vi "actuate_voltageStepExp_v0.05.vi"(0 "Phase Cluster":T4, 1 "valve Time Cluster":T3, 2 "Didn't Lift?":bool, 3 "data in":T5={"daq_ao 1"="Dev1/ao0", "daq_ai 1"="Dev1/ai0", "experiment day folder"=path "D:/DATA/8-27-15 save func testing/test.lvm", "Multiclamp init error"=0, "Multiclamp Handle Out"=0, "sampling rate (Hz)"=10000, "trial name"=""}, 5 "PhaseLetter":string, 7 "controls array in":refnum<vi>[](array[refnum]), 9 "time to wait for solution change (min)":dbl=2.5 min=0.0 step=0.01, 11 "error in":errorcluster, 12 "common cluster":T7, 13 "individual controls in":T6) -> (4 "output cluster":T1, 6 "protocol waveform":waveform(dbl)[](graph), 8 "jumptestMonitor":waveform(dbl)[](graph) caption="protocol response", 10 "control array out":refnum<vi>[](array[refnum]), 14 "experiment VI ref":refnum<vi>, 15 "error out":errorcluster)   [LabVIEW 2019]
uses:
  pipette cleaning/pressure box/cleaning_soft/controls/actuator_type.ctl
  pipette cleaning/pressure box/cleaning_soft/controls/actuator_cluster.ctl
  machine_vision/coordinate model vis/transform_properties_actuators.ctl
  machine_vision/controls/transform_cluster_actuator.ctl
  controls/NH_method.ctl
  pipette cleaning/pressure box/cleaning_soft/controls/pressure_box_type.ctl
  pipette cleaning/pressure box/cleaning_soft/controls/pressure_box_control.ctl
  multipatch/controls/multipatch_common_controls_v4.ctl
  controls/memtest_def.ctl
  multipatch/controls/multipatch_individual_controls_v5.ctl
  Controls/Data.ctl
panel:
  in  "VoltageStepValuesCluster":T2
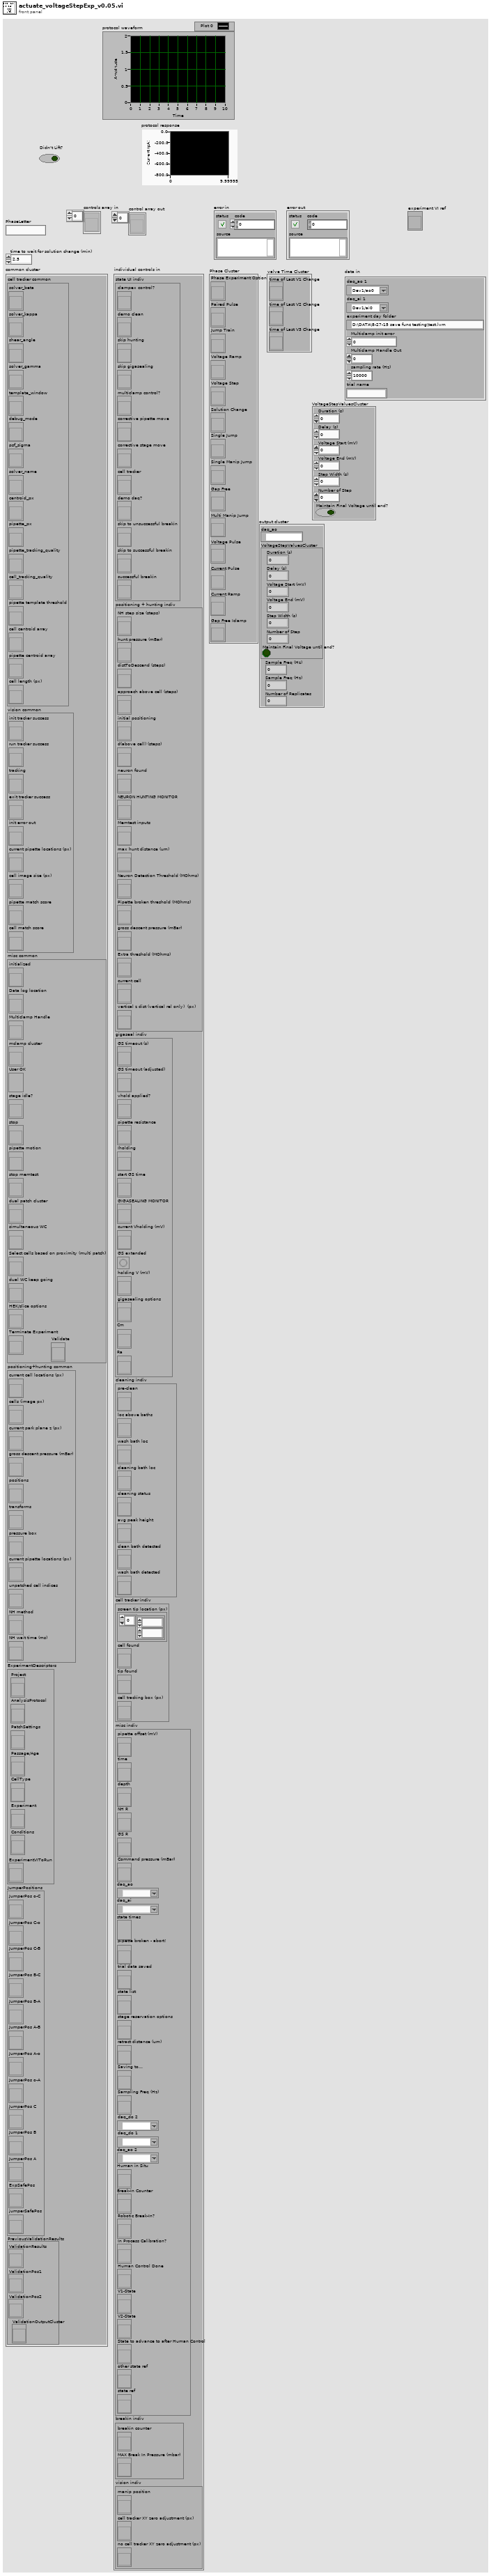
[diagram p1: front panel]
types:
  T1 = cluster{"daq_ao":tag, "VoltageStepValuesCluster":cluster{"Duration (s)":dbl, "Delay (s)":dbl, "Voltage Start (mV)":dbl, "Voltage End (mV)":dbl, "Step Width (s)":dbl, "Number of Step":dbl, "Maintain Final Voltage until end?":bool}, "Sample Freq (Hz)":dbl, "Sample Freq (Hz)":dbl, "Number of Replicates":i16}
  T2 = cluster{"Duration (s)":dbl, "Delay (s)":dbl, "Voltage Start (mV)":dbl, "Voltage End (mV)":dbl, "Step Width (s)":dbl, "Number of Step":dbl, "Maintain Final Voltage until end?":bool}
  T3 = cluster{"time of Last V1 Change":refnum<vi>, "time of Last V2 Change":refnum<vi>, "time of Last V3 Change":refnum<vi>}
  T4 = cluster{"Phase Experiment Option":refnum<vi>, "Paired Pulse":refnum<vi>, "Jump Train":refnum<vi>, "Voltage Ramp":refnum<vi>, "Voltage Step":refnum<vi>, "Solution Change":refnum<vi>, "Single Jump":refnum<vi>, "Single Manip Jump":refnum<vi>, "Gap Free":refnum<vi>, "Multi Manip Jump":refnum<vi>, "Voltage Pulse":refnum<vi>, "Current Pulse":refnum<vi>, "Current Ramp":refnum<vi>, "Gap Free Iclamp":refnum<vi>}
  T5 = typedef "Data.ctl" = cluster{"daq_ao 1":tag, "daq_ai 1":tag, "experiment day folder":path, "Multiclamp init error":i32, "Multiclamp Handle Out":u32, "sampling rate (Hz)":i32, "trial name":string}
  T6 = typedef "multipatch_individual_controls_v5.ctl" = cluster{"state UI indiv":cluster{"clampex control?":refnum<vi>, "demo clean":refnum<vi>, "skip hunting":refnum<vi>, "skip gigasealing":refnum<vi>, "multiclamp control?":refnum<vi>, "corrective pipette move":refnum<vi>, "corrective stage move":refnum<vi>, "cell tracker":refnum<vi>, "demo daq?":refnum<vi>, "skip to unsuccessful breakin":refnum<vi>, "skip to successful breakin":refnum<vi>, "successful breakin":refnum<vi>}, "positioning + hunting indiv":cluster{"NH step size (steps)":refnum<vi>, "hunt pressure (mBar)":refnum<vi>, "distToDescend (steps)":refnum<vi>, "approach above cell (steps)":refnum<vi>, "initial positioning":refnum<vi>, "d(above cell) (steps)":refnum<vi>, "neuron found":refnum<vi>, "NEURON HUNTING MONITOR":refnum<vi>, "Memtest inputs":refnum<vi>, "max hunt distance (um)":refnum<vi>, "Neuron Detection Threshold (MOhms)":refnum<vi>, "Pipette broken threshold (MOhms)":refnum<vi>, "gross descent pressure (mBar)":refnum<vi>, "Extra threshold (MOhms)":refnum<vi>, "current cell":refnum<vi>, "vertical z dist (vertical rel only)  (px)":refnum<vi>}, "gigaseal indiv":cluster{"GS timeout (s)":refnum<vi>, "GS timeout (adjusted)":refnum<vi>, "vhold applied?":refnum<vi>, "pipette resistance":refnum<vi>, "Iholding":refnum<vi>, "start GS time":refnum<vi>, "GIGASEALING MONITOR":refnum<vi>, "current Vholding (mV)":refnum<vi>, "GS extended":refnum<vi>, "holding V (mV)":refnum<vi>, "gigasealing options":refnum<vi>, "Cm":refnum<vi>, "Ra ":refnum<vi>}, "cleaning indiv":cluster{"pre-clean":refnum<vi>, "loc above baths":refnum<vi>, "wash bath loc":refnum<vi>, "cleaning bath loc":refnum<vi>, "cleaning status":refnum<vi>, "avg peak height":refnum<vi>, "clean bath detected":refnum<vi>, "wash bath detected":refnum<vi>}, "cell tracker indiv":cluster{"screen tip location (px)":refnum<vi>, "cell found":refnum<vi>, "tip found":refnum<vi>, "cell tracking box (px)":refnum<vi>}, "misc indiv":cluster{"pipette offset (mV)":refnum<vi>, "time":refnum<vi>, "depth":refnum<vi>, "NH R":refnum<vi>, "GS R":refnum<vi>, "Command pressure (mBar)":refnum<vi>, "daq_ao":tag, "daq_ai":tag, "state times":refnum<vi>, "pipette broken - abort!":refnum<vi>, "trial data saved":refnum<vi>, "state list":refnum<vi>, "stage reservation options":refnum<vi>, "retract distance (um)":refnum<vi>, "Saving to...":refnum<vi>, "Sampling Freq (Hz)":refnum<vi>, "daq_do 2":tag, "daq_do 1":tag, "daq_ao 2":tag, "Human in Situ":refnum<vi>, "Break-In Counter":refnum<vi>, "Robotic Break-In?":refnum<vi>, "In Process Calibration?":refnum<vi>, "Human Control Done":refnum<vi>, "V1-State":refnum<vi>, "V2-State":refnum<vi>, "State to advance to after Human Control":refnum<vi>, "other state ref":refnum<vi>, "state ref":refnum<vi>}, "breakin indiv":cluster{"breakin counter":refnum<vi>, "MAX Break In Pressure (mbar)":refnum<vi>}, "vision indiv":cluster{"manip position":refnum<vi>, "cell tracker XY zero adjustment (px)":refnum<vi>, "no cell tracker XY zero adjustment (px)":refnum<vi>}}
  T7 = typedef "multipatch_common_controls_v4.ctl" = cluster{"cell tracker common":cluster{"solver_beta":refnum<vi>, "solver_kappa":refnum<vi>, "shear_angle":refnum<vi>, "solver_gamma":refnum<vi>, "template_window":refnum<vi>, "debug_mode":refnum<vi>, "psf_sigma":refnum<vi>, "solver_name":refnum<vi>, "centroid_px":refnum<vi>, "pipette_px":refnum<vi>, "pipette_tracking_quality":refnum<vi>, "cell_tracking_quality":refnum<vi>, "pipette template threshold":refnum<vi>, "cell centroid array":refnum<vi>, "pipette centroid array":refnum<vi>, "cell length (px)":refnum<vi>}, "vision common":cluster{"init tracker success":refnum<vi>, "run tracker success":refnum<vi>, "tracking":refnum<vi>, "exit tracker success":refnum<vi>, "init error out":refnum<vi>, "current pipette locations (px)":refnum<vi>, "cell image size (px)":refnum<vi>, "pipette match score":refnum<vi>, "cell match score":refnum<vi>}, "misc common":cluster{"initialized":refnum<vi>, "Data log location":refnum<vi>, "Multiclamp Handle":refnum<vi>, "mclamp cluster":refnum<vi>, "User OK":refnum<vi>, "stage idle?":refnum<vi>, "stop":refnum<vi>, "pipette motion":refnum<vi>, "stop memtest":refnum<vi>, "dual patch cluster":refnum<vi>, "simultaneous WC":refnum<vi>, "Select cells based on proximity (multi patch)":refnum<vi>, "dual WC keep going":refnum<vi>, "HEK/slice options":refnum<vi>, "Terminate Experiment":refnum<vi>, "Validate":refnum<vi>}, "positioning+hunting common":cluster{"current cell locations (px)":refnum<vi>, "cells (image px)":refnum<vi>, "current park plane z (px)":refnum<vi>, "gross descent pressure (mBar)":refnum<vi>, "positions":refnum<vi>, "transforms":refnum<vi>, "pressure box":refnum<vi>, "current pipette locations (px)":refnum<vi>, "unpatched cell indices":refnum<vi>, "NH method":refnum<vi>, "NH wait time (ms)":refnum<vi>}, "ExperimentDescriptors":cluster{"Project":refnum<vi>, "AnalysisProtocol":refnum<vi>, "PatchSettings":refnum<vi>, "Passage/Age":refnum<vi>, "CellType":refnum<vi>, "Experiment":refnum<vi>, "Conditions":refnum<vi>, "ExperimentVIToRun":refnum<vi>}, "JumperPositions":cluster{"JumperPos o-C":refnum<vi>, "JumperPos C-o":refnum<vi>, "JumperPos C-B":refnum<vi>, "JumperPos B-C":refnum<vi>, "JumperPos B-A":refnum<vi>, "JumperPos A-B":refnum<vi>, "JumperPos A-o":refnum<vi>, "JumperPos o-A":refnum<vi>, "JumperPos C":refnum<vi>, "JumperPos B":refnum<vi>, "JumperPos A":refnum<vi>, "ExpSafePos":refnum<vi>, "jumperSafePos":refnum<vi>}, "PreviousValidationResults":cluster{"ValidationResults":refnum<vi>, "ValidationPos1":refnum<vi>, "ValidationPos2":refnum<vi>, "ValidationOutputCluster":refnum<vi>}}
  T8 = cluster{"Which Position to use for Experiment":enum16{"Jumper Safe Position", "Experiment Safe Position", "Jumper Position A", "Jumper Position B", "Jumper Position C", "Jumper Position o-A", "Jumper Position A-o", "Jumper Position A-B", "Jumper Position B-A", "Jumper Position B-C", "Jumper Position C-B", "Jumper Position C-o", "Jumper Position o-C", "Don't Move"}, "Duration (s)":dbl, "Delay (s)":dbl, "Step Width (s)":dbl, "Voltage Start (mV)":dbl, "Voltage Step (mV)":dbl, "Replicates":dbl, "Voltage End (mV)":dbl, "Number of Step":dbl, "Vholding (mV)":dbl, "Valve 1 Position":i16, "Valve 2 Position":i16, "Valve 3 Position":i16, "valve 1 used now?":bool, "valve 2 used now?":bool, "valve 3 used now? ":bool, "Total Step Time (s)":dbl, "Maintain Final Voltage until end?":bool, "protocol Preview":waveform(dbl)[]}
  T9 = enum16{"Jumper Safe Position", "Experiment Safe Position", "Jumper Position A", "Jumper Position B", "Jumper Position C", "Jumper Position o-A", "Jumper Position A-o", "Jumper Position A-B", "Jumper Position B-A", "Jumper Position B-C", "Jumper Position C-B", "Jumper Position C-o", "Jumper Position o-C", "Don't Move"}
  T10 = enum16{"manipulator 1", "manipulator 2", "manipulator 3", "manipulator 4"}
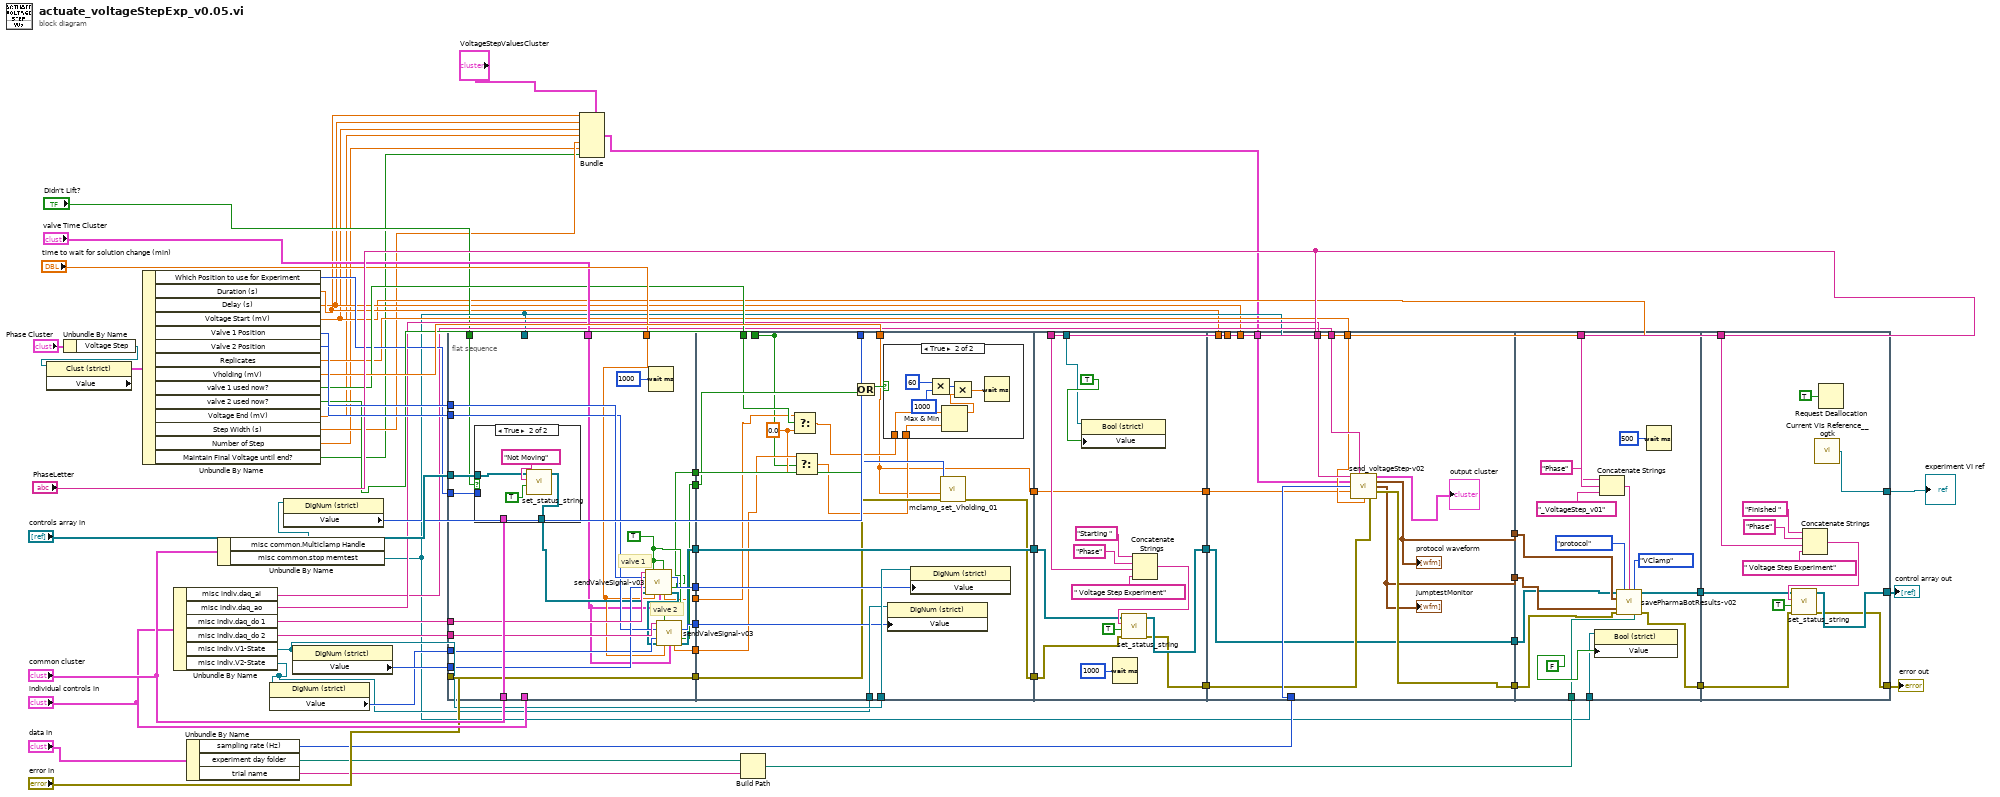
[diagram p0: block diagram]
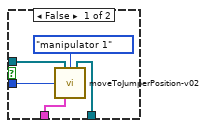
[diagram p2: hidden frame]
diagram:
  n1 = Unbundle By Name("Phase Cluster") -> ("Voltage Step"=w44:refnum<vi>)
  n2 = property class="Clust (strict)"(reference=w44) -> ("Value"=w43:T8)  [unwired: 1 in, 2 out]
  n3 = Unbundle By Name(w43) -> ("Which Position to use for Experiment"=w19:T9, "Duration (s)"=w12:dbl, "Delay (s)"=w11:dbl, "Voltage Start (mV)"=w10:dbl, "Valve 1 Position"=w42:i16, "Valve 2 Position"=w41:i16, "Replicates"=w18:dbl, "Vholding (mV)"=w28:dbl, "valve 1 used now?"=w21:bool, "valve 2 used now?"=w20:bool, "Voltage End (mV)"=w9:dbl, "Step Width (s)"=w8:dbl, "Number of Step"=w4:dbl, "Maintain Final Voltage until end?"=w3:bool)
  n4 = Unbundle By Name("individual controls in") -> ("misc indiv.daq_ai"=w15:tag, "misc indiv.daq_ao"=w16:tag, "misc indiv.daq_do 1"=w64:tag, "misc indiv.daq_do 2"=w63:tag, "misc indiv.V1-State"=w55:refnum<vi>, "misc indiv.V2-State"=w54:refnum<vi>)
  n5 = Unbundle By Name("data in") -> ("sampling rate (Hz)"=w17:i32, "experiment day folder"=w48:path, "trial name"=w47:string)
  n6 = Unbundle By Name("common cluster") -> ("misc common.Multiclamp Handle"=w27:refnum<vi>, "misc common.stop memtest"=w14:refnum<vi>)
  n7 = property class="DigNum (strict)"(reference=w54) -> ("Value"=w56:u16)  [unwired: 1 in, 2 out]
  n8 = property class="DigNum (strict)"(reference=w27) -> ("Value"=w26:u32)  [unwired: 1 in, 2 out]
  n9 = property class="DigNum (strict)"(reference=w55) -> ("Value"=w57:u16)  [unwired: 1 in, 2 out]
  n10 = flat-sequence {
    tunnel: "common cluster" -> [w89]
    tunnel: "individual controls in" -> [_]
    tunnel: [w86] -> w59
    tunnel: [w83] -> w53
    tunnel: [w82] -> w52
    tunnel: [w76] -> w35
    tunnel: [w74] -> w30
    tunnel: [w73] -> w29
    tunnel: "time to wait for solution change (min)" -> [w72]
    tunnel: "valve Time Cluster" -> [w71]
    tunnel: [w70] -> w23
    tunnel: [w69] -> w22
    tunnel: w14 -> [_]
    tunnel: "Didn't Lift?" -> [w67]
    tunnel: w19 -> [w90]
    tunnel: w64 -> [w88]
    tunnel: w63 -> [w87]
    tunnel: "error in" -> [w86]
    tunnel: w57 -> [w85]
    tunnel: w56 -> [w84]
    tunnel: w42 -> [w81]
    tunnel: w41 -> [w80]
    tunnel: "controls array in" -> [w79]
    tunnel: [w108] -> w60
    tunnel: w59 -> [w110]
    tunnel: w55 -> [w118]
    tunnel: w54 -> [w117]
    tunnel: w53 -> [w116]
    tunnel: w52 -> [w115]
    tunnel: [w114] -> w36
    tunnel: w35 -> [w114]
    tunnel: w30 -> [w112]
    tunnel: w29 -> [w111]
    tunnel: w28 -> [w100]
    tunnel: w26 -> [w109]
    tunnel: w23 -> [w105]
    tunnel: w22 -> [w104]
    tunnel: w21 -> [w106]
    tunnel: [w101] -> _
    tunnel: w20 -> [w101]
    tunnel: [w100] -> w5
    tunnel: w14 -> [w127]
    tunnel: [w129] -> w61
    tunnel: w60 -> [w130]
    tunnel: [w131] -> w37
    tunnel: w36 -> [w132]
    tunnel: "PhaseLetter" -> [w133]
    tunnel: [w126] -> w6
    tunnel: w5 -> [w126]
    tunnel: w15 -> [w151]
    tunnel: w16 -> [w150]
    tunnel: w61 -> [w145]
    tunnel: [w148] -> w51
    tunnel: [w142] -> w50
    tunnel: w18 -> [w146]
    tunnel: w12 -> [_]
    tunnel: w17 -> [w147]
    tunnel: w10 -> [_]
    tunnel: w11 -> [_]
    tunnel: [w144] -> w40
    tunnel: [w143] -> w38
    tunnel: w37 -> [w143]
    tunnel: w7 -> [w141]
    tunnel: w6 -> [w140]
    tunnel: w14 -> [w166]
    tunnel: w51 -> [w165]
    tunnel: w50 -> [w164]
    tunnel: w46 -> [w161]
    tunnel: "PhaseLetter" -> [w159]
    tunnel: w40 -> [w156]
    tunnel: w38 -> [w155]
    tunnel: [w153] -> w33
    tunnel: [w154] -> w32
    tunnel: [w173] -> w34
    tunnel: [w172] -> w58
    tunnel: w33 -> [w171]
    tunnel: w32 -> [w174]
    tunnel: "PhaseLetter" -> [w170]
    tunnel: [w169] -> w1
    frame #0 {
      w75 = TRUE ("Set Status")
      # "valve 2"
      # "valve 1"
      n11 = case shown="True" w67 {
        tunnel: w90 -> [w95 _]
        tunnel: w89 -> [w94 _]
        tunnel: w79 -> [w92 w96]
        tunnel: [w91 w97] -> w78
        frame False {
          n12 = call "moveToJumperPosition-v02.vi"("which manipulator"=T10."manipulator 1", "controls array in"=w92, "Which Jumper Position to move to?"=w95, "common cluster"=w94) -> ("control array out"=w91:refnum<vi>[])  [unwired: 10 in, 1 out]
        }
        frame True {
          n13 = call "set_status_string.vi"("new line?"=TRUE, "status string in"="Not Moving", "controls array"=w96) -> ("controls array out"=w97:refnum<vi>[])  [unwired: 7 in, 1 out]
        }
      }
      n14 = call "sendValveSignal-v03.vi"("daq_do"=w88, "Set Status"=w75, "Valve1?"=w75, "ChangeToValve"=w81, "CurrentValve"=w85, "controls array in"=w78, "time to wait for solution change (min)"=w72, "valve Time Cluster"=w71) -> ("ValveSetTo"=w82:u16, "valve changed?"=w74:bool, "additional time to wait (min)"=w70:dbl, "control array out"=w77:refnum<vi>[])  [unwired: 4 in]
      n15 = Wait (ms)(milliseconds to wait=u32 1000) -> ()  [unwired: 1 out]
      n16 = call "sendValveSignal-v03.vi"("daq_do"=w87, "Set Status"=w75, "ChangeToValve"=w80, "CurrentValve"=w84, "controls array in"=w77, "time to wait for solution change (min)"=w72, "valve Time Cluster"=w71) -> ("ValveSetTo"=w83:u16, "valve changed?"=w73:bool, "additional time to wait (min)"=w69:dbl, "control array out"=w76:refnum<vi>[])  [unwired: 5 in]
    }
    frame #1 {
      w102 = 0.0 ("f")
      n17 = Select(t=w105, s=w106, f=w102) -> (s? t:f=w107:dbl)
      n18 = Select(t=w104, s=w101, f=w102) -> (s? t:f=w103:dbl)
      n19 = Or(x=w112, y=w111) -> (x .or. y?=w113:bool)
      n20 = case shown="True" w113 {
        tunnel: w107 -> [_ w121]
        tunnel: w103 -> [_ w120]
        frame False {
        }
        frame True {
          n21 = Multiply(x=u32 60 ("milliseconds to wait"), y=u32 1000) -> (x*y=w123:u32)
          n22 = Max & Min(x=w121, y=w120) -> (max(x,y)=w119:dbl)  [unwired: 1 out]
          n23 = Multiply(x=w123, y=w119) -> (x*y=w122:dbl)
          n24 = Wait (ms)(milliseconds to wait=w122) -> ()  [unwired: 1 out]
        }
      }
      n25 = property class="DigNum (strict)"(reference=w117, "Value"=w116) -> ()  [unwired: 1 in, 2 out]
      n26 = property class="DigNum (strict)"(reference=w118, "Value"=w115) -> ()  [unwired: 1 in, 2 out]
      n27 = call "mclamp_set_Vholding_01.vi"("error in (no error)"=w110, "set holding (mV)"=w100, "Multiclamp Handle Out"=w109) -> ("error out"=w108:errorcluster)  [unwired: 7 in, 1 out]
    }
    frame #2 {
      n28 = property class="Bool (strict)"(reference=w127, "Value"=TRUE ("stop memtest")) -> ()  [unwired: 1 in, 2 out]
      n29 = Wait (ms)(milliseconds to wait=u32 1000) -> ()  [unwired: 1 out]
      n30 = Concatenate Strings("Starting " ("string"), "Phase" ("string"), w133, " Voltage Step Experiment" ("string")) -> (w135:string)
      n31 = call "set_status_string.vi"("error in"=w130, "new line?"=TRUE, "status string in"=w135, "controls array"=w132) -> ("error out"=w129:errorcluster, "controls array out"=w131:refnum<vi>[])  [unwired: 6 in]
    }
    frame #3 {
      n32 = call "send_voltageStep-v02.vi"("daq_ao"=w150, "daq_ai"=w151, "VoltageStepValuesCluster"=w141, "Sample Freq (Hz)"=w147, "set holding (mV)"=w140, "Number of Replicates"=w146, "error in"=w145) -> ("output cluster"=→"output cluster":T1, "output waveform"=w148:waveform(dbl)[], "protocol response"=w142:waveform(dbl)[], "error out"=w144:errorcluster)  [unwired: 5 in]
      "jumptestMonitor" <- w142
      "protocol waveform" <- w148
    }
    frame #4 {
      n33 = property class="Bool (strict)"(reference=w166, "Value"=FALSE ("stop memtest")) -> ()  [unwired: 1 in, 2 out]
      n34 = Concatenate Strings("Phase" ("string"), w159, "_VoltageStep_v01" ("string")) -> (w160:string)
      n35 = call "savePharmaBotResults-v02.vi"("controls array"=w155, "protocol or memtest"=enum16{"protocol", "memtest", "validation"}."protocol", "ExpPhase"=w160, "which clamp"=enum16{"VClamp", "IClamp"}."VClamp", "protocol waveform"=w165, "protocol response"=w164, "error in"=w156, "Save to (folder dir)"=w161) -> ("controls array out"=w154:refnum<vi>[], "error out"=w153:errorcluster)  [unwired: 6 in]
      n36 = Wait (ms)(milliseconds to wait=u32 500) -> ()  [unwired: 1 out]
    }
    frame #5 {
      n37 = Concatenate Strings("Finished " ("string"), "Phase" ("string"), w170, " Voltage Step Experiment" ("string")) -> (w176:string)
      n38 = call "set_status_string.vi"("error in"=w171, "new line?"=TRUE, "status string in"=w176, "controls array"=w174) -> ("error out"=w172:errorcluster, "controls array out"=w173:refnum<vi>[])  [unwired: 6 in]
      n39 = call "Current VIs Reference__ogtk.vi"() -> ("Current VI's reference"=w169:refnum<vi>)  [unwired: 5 in]
      n40 = Request Deallocation(TRUE ("flag")) -> ()
    }
  }
  n41 = Bundle(cluster="VoltageStepValuesCluster", "Duration (s)"=w12, "Delay (s)"=w11, "Voltage Start (mV)"=w10, "Voltage End (mV)"=w9, "Step Width (s)"=w8, "Number of Step"=w4, "Maintain Final Voltage until end?"=w3) -> (w7:T2)
  n42 = Build Path(base path=w48, name or relative path=w47) -> (appended path=w46:path)
  "error out" <- w58
  "control array out" <- w34
  "experiment VI ref" <- w1
